vi "Last_modified_date.vi"(0 "Update Now":bool) -> (1 "RevisionString":string)   [LabVIEW 2015]
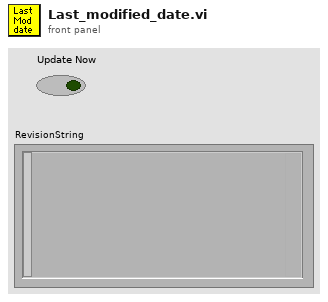
[diagram p1: front panel]
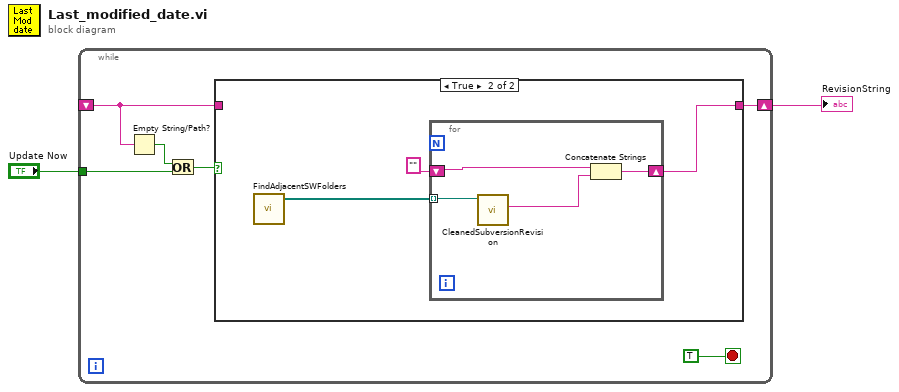
[diagram p0: block diagram]
diagram:
  n1 = while {
    shift-right: [w8] -> w1
    shift-left: _ -> [w4]
    tunnel: "Update Now" -> [w5]
    stop <- TRUE stop-if-true
    n2 = Empty String/Path?(string/path=w4) -> (empty?=w3:bool)
    n3 = Or(x=w3, y=w5) -> (x .or. y?=w6:bool)
    n4 = case shown="True" w6 {
      tunnel: [w9 w11] -> w8
      tunnel: w4 -> [w9 _]
      frame False {
      }
      frame True {
        n5 = call "FindAdjacentSWFolders.vi"() -> ("Array"=w12:path[])  [unwired: 11 in]
        n6 = for {
          tunnel: w12 -> [w16] mode=indexing
          shift-right: [w14] -> w11
          shift-left: "" ("CleanRevisionString") -> [w13]
          n7 = call "CleanedSubversionRevision.vi"("File Path Control"=w16) -> ("CleanRevisionString"=w15:string)  [unwired: 9 in, 1 out]
          n8 = Concatenate Strings(w13, w15) -> (w14:string)
        }
      }
    }
  }
  "RevisionString" <- w1
